vi "medicaoIXV.vi"() -> ()   [LabVIEW 2012]
uses:
  <vilib>/Utility/file.llb/Write To Spreadsheet File (string).vi
  <vilib>/Utility/file.llb/Write To Spreadsheet File (DBL).vi
  <instrlib>/Agilent 6XXX Series/Agilent 6XXX Series.lvlib
panel:
  out "reset graph":bool=TRUE
  out "tabela":dbl[][](array[numeric])
  in  "Tab Control":enum32{"Entrada de dados", "Saída de dados"}(tab)
  in  "Irradiância":dbl caption="Irradiância(W/cm²)"
  in  "T.J":dbl caption="Tensão\ndo joelho"
  in  "p.a.j":dbl caption="Pontos antes\ndo joelho"
  in  "nMedições":i16=1 caption="N° curvas" min=1
  in  "area":dbl caption="Área da célula(cm²)"
  in  "Tipo":string caption="Tipo da célula"
  in  "Formato":u16(ring) items=[".txt", ".csv"]
  out "ON/OFF1":bool caption="ON/OFF"
  in  "p.d.j":dbl caption="Pontos depois\ndo joelho"
  in  "T.M":dbl caption="Tensão máxima"
  in  "Nome da célula":string
  in  "Local":path
  in  "Delay(ms)":dbl
  in  "Start":bool
  in  "temperatura":dbl caption="Temperatura da célula"
  out "Eficiência":dbl caption="Eficiência(%)"
  out "FF":dbl
  in  "stopProgram":bool caption="Parar Programa"
  out "Imp":dbl caption="Imp(A)"
  out "Vmp":dbl caption="Vmp(V)"
  out "Pmp":dbl caption="Pmp(W)"
  out "Icc":dbl caption="Icc (A)"
  out "Vca":dbl caption="Vca (V)"
  in  "Print Screen":bool
  out "IXV":cluster{"Y":dbl[], "Y":dbl[]}[](graph)
  out "output voltage":dbl
  out "Tensao Atual (V)":dbl
  out "Corrente Atual\n(A)":dbl
  out "Ponto Atual":i32
  out "tabela":dbl[][](array[numeric]) caption="TABELA DE DADOS\nTensão(Fonte)      Pontos             Tensao           Corrente" format="%0.8f"
  in  "stop":bool caption="Parar Medição"
  out "ON/OFF2":bool caption="ON/OFF"
  out "tempoMedicao":dbl caption="Tempo de medicao do ponto(s)"
  in  "CorrenteGraph":dbl
  in  "TensaoGraph":dbl
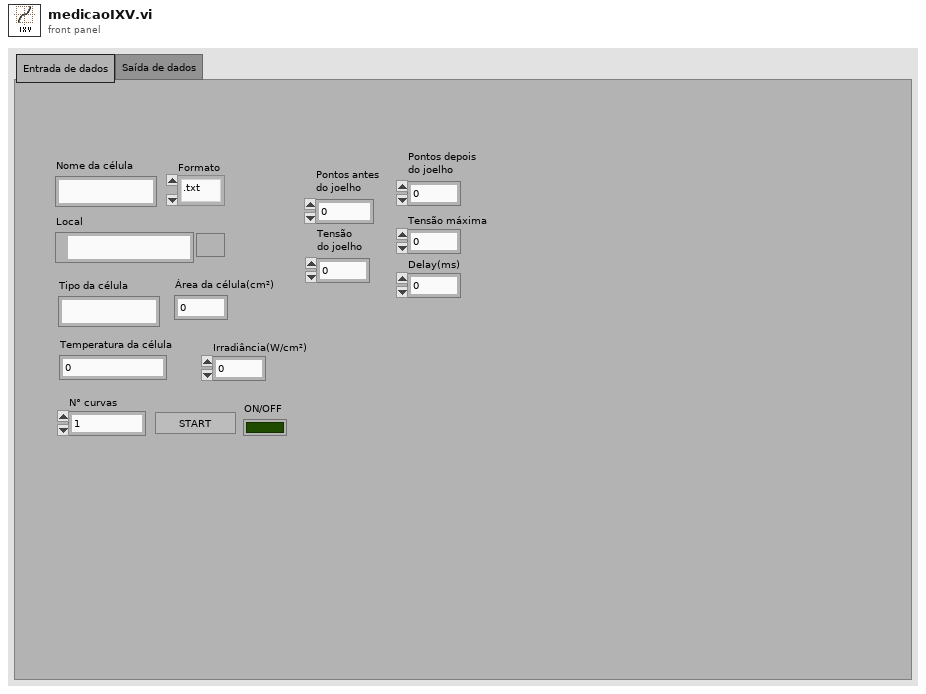
[diagram p1: front panel]
types:
  T1 = typedef "imagedata.ctl" = cluster{"image type":i32, "image depth":i32, "image":u8[], "mask":u8[], "colors":u32[], "Rectangle":cluster{"left":i16, "top":i16, "right":i16, "bottom":i16}}
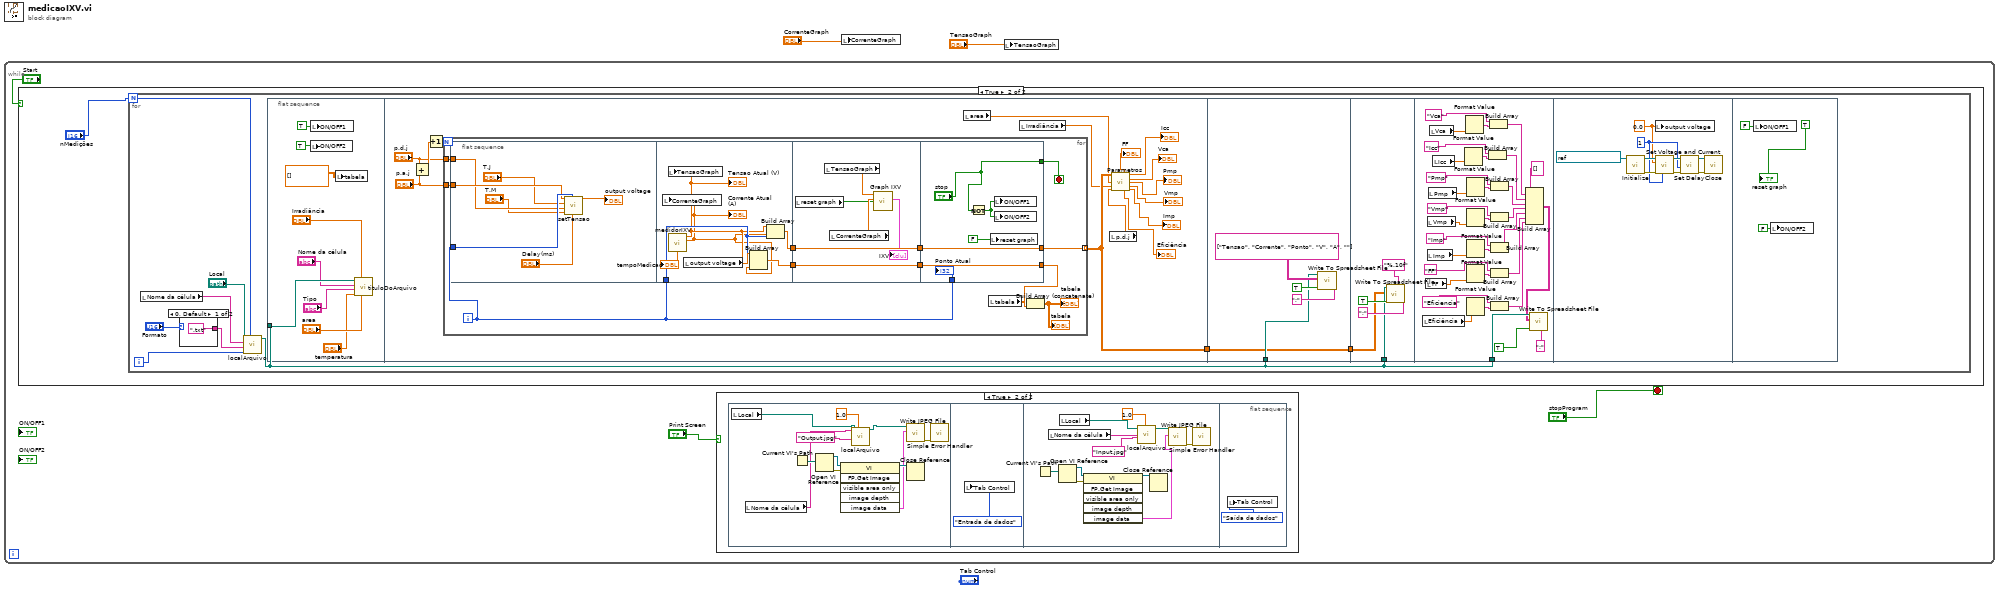
[diagram p0: block diagram]
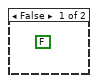
[diagram p3: hidden frame]
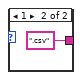
[diagram p4: hidden frame]
diagram:
  n1 = while {
    stop <- "stopProgram" stop-if-true
    n2 = case shown="True" "Start" {
      frame False {
        (unwired) FALSE
      }
      frame True {
        n3 = for {
          N: "nMedições" -> [w36]
          i -> [w32]
          n4 = local read "Nome da célula"() -> (w34:string)
          n5 = case shown="0, Default" "Formato" {
            tunnel: [".txt" ".csv"] -> w33
            frame 0, Default {
            }
            frame 1 {
            }
          }
          n6 = call "localArquivo.vi"("quantidadeDeArquivos"=w36, "numeroDoArquivo"=w32, "extensão"=w33, "Nome do arquivo"=w34, "Local"="Local") -> ("Path"=w31:path)  [unwired: 6 in]
          n7 = flat-sequence {
            tunnel: w31 -> [w50]
            tunnel: [w65] -> w39
            tunnel: w31 -> [w105]
            tunnel: [w104] -> w38
            tunnel: w39 -> [w104]
            tunnel: w31 -> [w110]
            tunnel: w38 -> [w109]
            tunnel: w31 -> [w124]
            frame #0 {
              n8 = local write "ON/OFF2"(TRUE ("ON/OFF2")) -> ()
              n9 = local write "ON/OFF1"(TRUE ("ON/OFF")) -> ()
              n10 = local write "tabela"(dbl[][] [] ("array")) -> ()
              n11 = call "tituloDoArquivo.vi"("area"="area", "irradiancia"="Irradiância", "temperatura"="temperatura", "Tipo"="Tipo", "Nome da célula"="Nome da célula", "file path (dialog if empty)"=w50) -> ()  [unwired: 6 in]
            }
            frame #1 {
              n12 = Add(x="p.d.j", y="p.a.j") -> (x+y=w57:dbl)
              n13 = Increment(x=w57) -> (x+1=w64:dbl)
              n14 = for {
                N: w64 -> [_]
                tunnel: [w77] -> w65 mode=indexing
                tunnel: "p.a.j" -> [w67]
                tunnel: "p.d.j" -> [w66]
                i -> [w71]
                stop <- w70 stop-if-true
                n15 = flat-sequence {
                  tunnel: w71 -> [w83]
                  tunnel: w67 -> [w81]
                  tunnel: w66 -> [w80]
                  tunnel: w71 -> [w87]
                  tunnel: [w90] -> w76
                  tunnel: [w91] -> w75
                  tunnel: [w97] -> w69
                  tunnel: [w96] -> w68
                  tunnel: w75 -> [w96]
                  tunnel: w76 -> [w97]
                  tunnel: [w102] -> w74
                  tunnel: [w103] -> w77
                  tunnel: w69 -> [w103]
                  tunnel: w68 -> [w102]
                  tunnel: w71 -> [w101]
                  tunnel: ["stop"] -> w70
                  frame #0 {
                    n16 = call "setTensao.vi"("delay(ms)"="Delay(ms)", "Ponto atual"=w83, "T.M"="T.M", "P.D.J"=w80, "T.J"="T.J", "P.A.J"=w81) -> ("output voltage"=→"output voltage":dbl)  [unwired: 5 in]
                  }
                  frame #1 {
                    n17 = call "medidorIXV.vi"() -> ("tempo de medicao"=→"tempoMedicao":dbl, "Corrente Atual"=w85:dbl, "Tensao Atual"=w86:dbl)  [unwired: 9 in]
                    "Corrente Atual\n(A)" <- w85
                    "Tensao Atual (V)" <- w86
                    n18 = local write "CorrenteGraph"(w85) -> ()
                    n19 = local write "TensaoGraph"(w86) -> ()
                    n20 = local read "output voltage"() -> (w88:dbl)
                    n21 = Build Array(w88, w87, w86, w85) -> (w91:dbl[])
                    n22 = Build Array(w86, w85, w87) -> (w90:dbl[])
                  }
                  frame #2 {
                    n23 = local read "reset graph"() -> (w92:bool)
                    n24 = local read "TensaoGraph"() -> (w95:dbl)
                    n25 = local read "CorrenteGraph"() -> (w94:dbl)
                    n26 = call "Graph IXV"("Reset"=w92, "Y Input"=w94, "X Input"=w95) -> ("XY Graph"=→"IXV":cluster{"Y":dbl[], "Y":dbl[]}[])  [unwired: 2 in, 6 out]
                  }
                  frame #3 {
                    n27 = Not(x="stop") -> (.not. x?=w99:bool)
                    n28 = local write "reset graph"(FALSE) -> ()
                    n29 = local write "ON/OFF1"(w99) -> ()
                    n30 = local write "ON/OFF2"(w99) -> ()
                    "Ponto Atual" <- w101
                  }
                }
                n31 = local read "tabela"() -> (w73:dbl[][])
                n32 = Build Array (concatenate)(w73, w74) -> (→"tabela" →"tabela":dbl[][])
              }
              n33 = local read "area"() -> (w53:dbl)
              n34 = local read "Irradiância"() -> (w52:dbl)
              n35 = local read "p.d.j"() -> (w63:dbl)
              n36 = call "Parametros.vi"("VetorDeDados"=w65, "area"=w53, "irradiancia"=w52, "pontos"=w63) -> ("FF"=→"FF":dbl, "Icc"=→"Icc":dbl, "Vca"=→"Vca":dbl, "Pmp"=→"Pmp":dbl, "Vmp"=→"Vmp":dbl, "eficiencia"=→"Eficiência":dbl, "Imp"=→"Imp":dbl)  [unwired: 5 in]
            }
            frame #2 {
              n37 = call-poly <vilib>:"Write To Spreadsheet File.vi"("delimiter (\\t)"=";" ("delimiter (\\t)"), "append to file? (new file:F)"=TRUE, "2D data"=string[][] [["Tensao", "Corrente", "Ponto"], ["V", "A", ""]], "file path (dialog if empty)"=w105) -> ()  [unwired: 4 in, 1 out]
            }
            frame #3 {
              n38 = call-poly <vilib>:"Write To Spreadsheet File.vi"("delimiter (\\t)"=";" ("delimiter (\\t)"), "format (%.3f)"="%.10f", "append to file? (new file:F)"=TRUE, "2D data"=w109, "file path (dialog if empty)"=w110) -> ()  [unwired: 3 in, 1 out]
            }
            frame #4 {
              n39 = local read "Eficiência"() -> (w117:dbl)
              n40 = local read "FF"() -> (w118:dbl)
              n41 = local read "Vmp"() -> (w138:dbl)
              n42 = local read "Imp"() -> (w139:dbl)
              n43 = local read "Pmp"() -> (w137:dbl)
              n44 = local read "Vca"() -> (w126:dbl)
              n45 = local read "Icc"() -> (w136:dbl)
              n46 = Format Value(value (0)=w136) -> (output string=w129:string)  [unwired: 2 in]
              n47 = Format Value(value (0)=w126) -> (output string=w127:string)  [unwired: 2 in]
              n48 = Format Value(value (0)=w137) -> (output string=w131:string)  [unwired: 2 in]
              n49 = Format Value(value (0)=w139) -> (output string=w135:string)  [unwired: 2 in]
              n50 = Format Value(value (0)=w138) -> (output string=w133:string)  [unwired: 2 in]
              n51 = Format Value(value (0)=w118) -> (output string=w123:string)  [unwired: 2 in]
              n52 = Format Value(value (0)=w117) -> (output string=w122:string)  [unwired: 2 in]
              n53 = Build Array("Icc", w129) -> (w141:string[])
              n54 = Build Array("Vca", w127) -> (w140:string[])
              n55 = Build Array("Pmp", w131) -> (w142:string[])
              n56 = Build Array("Imp", w135) -> (w144:string[])
              n57 = Build Array("Vmp", w133) -> (w143:string[])
              n58 = Build Array("FF" ("element"), w123) -> (w116:string[])
              n59 = Build Array("Eficiencia" ("element"), w122) -> (w115:string[])
              n60 = Build Array(string[] [] ("element"), w140, w141, w142, w143, w144, w116, w115) -> (w121:string[][])
              n61 = call-poly <vilib>:"Write To Spreadsheet File.vi"("delimiter (\\t)"=";" ("delimiter (\\t)"), "append to file? (new file:F)"=TRUE, "2D data"=w121, "file path (dialog if empty)"=w124) -> ()  [unwired: 4 in, 1 out]
            }
            frame #5 {
              w147 = 0.0 ("voltage (0 V)")
              w150 = u8 1 ("channel (1)")
              n62 = call <instrlib>:"Initialize.vi"("VISA resource name"=refnum<visa-resource-name> "GPIB0::5::INSTR") -> ("error out"=w152:errorcluster, "VISA resource name out"=w151:refnum<visa-resource-name>)  [unwired: 9 in]
              n63 = local write "output voltage"(w147) -> ()
              n64 = call <instrlib>:"Set Voltage and Current.vi"("channel (1)"=w150, "error in (no error)"=w152, "voltage (0 V)"=w147, "VISA resource name"=w151) -> ("error out"=w153:errorcluster, "VISA resource name out"=w154:refnum<visa-resource-name>)  [unwired: 6 in]
              n65 = call <instrlib>:"Set Delay.vi"("error in (no error)"=w153, "channel (1)"=w150, "VISA resource name"=w154) -> ("error out"=w148:errorcluster, "VISA resource name out"=w149:refnum<visa-resource-name>)  [unwired: 7 in]
              n66 = call <instrlib>:"Close.vi"("error in (no error)"=w148, "VISA resource name"=w149) -> ()  [unwired: 9 in, 1 out]
            }
            frame #6 {
              n67 = local write "ON/OFF1"(FALSE) -> ()
              n68 = local write "ON/OFF2"(FALSE ("ON/OFF")) -> ()
              "reset graph" <- TRUE
            }
          }
        }
      }
    }
    n69 = case shown="True" "Print Screen" {
      frame False {
      }
      frame True {
        n70 = flat-sequence {
          frame #0 {
            n71 = local read "Local"() -> (w9:path)
            n72 = local read "Nome da célula"() -> (w7:string)
            n73 = Current VI's Path() -> (path=w14:path)
            n74 = Open VI Reference(vi path=w14) -> (vi reference=w15:refnum<vi>, error out=w16:errorcluster)  [unwired: 5 in]
            n75 = invoke class="VI" method="FP.Get Image"(reference=w15, error in=w16) -> (reference out=w13:refnum<vi>, "image data"=w12:T1)  [unwired: 4 in, 4 out]
            n76 = call "localArquivo.vi"("quantidadeDeArquivos"=1.0, "extensão"="Output.jpg", "Nome do arquivo"=w7, "Local"=w9) -> ("Path"=w6:path)  [unwired: 7 in]
            n77 = call <vilib>:"Write JPEG File.vi"("image data"=w12, "path to JPEG file"=w6) -> ("error out"=w11:errorcluster)  [unwired: 8 in, 1 out]
            n78 = Close Reference(reference=w13) -> ()  [unwired: 1 in, 1 out]
            n79 = call <vilib>:"Simple Error Handler.vi"("error in (no error)"=w11) -> ()  [unwired: 4 in, 5 out]
          }
          frame #1 {
            n80 = local write "Tab Control"(enum32{"Entrada de dados", "Saída de dados"}."Entrada de dados" ("Tab Control")) -> ()
          }
          frame #2 {
            n81 = Current VI's Path() -> (path=w27:path)
            n82 = local read "Nome da célula"() -> (w21:string)
            n83 = Open VI Reference(vi path=w27) -> (vi reference=w26:refnum<vi>, error out=w25:errorcluster)  [unwired: 5 in]
            n84 = local read "Local"() -> (w20:path)
            n85 = invoke class="VI" method="FP.Get Image"(reference=w26, error in=w25) -> (reference out=w28:refnum<vi>, "image data"=w23:T1)  [unwired: 4 in, 4 out]
            n86 = call "localArquivo.vi"("quantidadeDeArquivos"=1.0, "extensão"="Input.jpg", "Nome do arquivo"=w21, "Local"=w20) -> ("Path"=w19:path)  [unwired: 7 in]
            n87 = Close Reference(reference=w28) -> ()  [unwired: 1 in, 1 out]
            n88 = call <vilib>:"Write JPEG File.vi"("image data"=w23, "path to JPEG file"=w19) -> ("error out"=w24:errorcluster)  [unwired: 8 in, 1 out]
            n89 = call <vilib>:"Simple Error Handler.vi"("error in (no error)"=w24) -> ()  [unwired: 4 in, 5 out]
          }
          frame #3 {
            n90 = local write "Tab Control"(enum32{"Entrada de dados", "Saída de dados"}."Saída de dados" ("Tab Control")) -> ()
          }
        }
      }
    }
  }
  n91 = local write "CorrenteGraph"("CorrenteGraph") -> ()
  n92 = local write "TensaoGraph"("TensaoGraph") -> ()
